vi "diffusion_sub.vi"(0 "X":dbl[](array[numeric]) format="%.2f", 1 "Standard Deviation":dbl[](array[numeric]) format="%.2f", 5 "Y":dbl[](array[numeric]) format="%.2f", 9 "Initial Guess Coefficients":dbl[](array[numeric])=[0.0, 1e-09, 0.0001, 0.8, 0.5] format="%.2e", 11 "max iteration":i32=200, 12 "Substitution Rules":T2(array[cluster])) -> (3 "Covariance":dbl[][](array[numeric]) format="%.2f", 4 "Best Fit Coefficients":dbl[](array[numeric]) format="%.2e", 6 "Best Fit":dbl[](array[numeric]) format="%.2f", 8 "ticks":i32=1, 10 "mse":dbl=nan format="%.2e", 14 "error":i32=-23033, 15 "model description":T1={"model"="b*(1+a*exp(-x/t1))/(1+x/t2)*(1+x/(4*t2))^(-1/2)+o", "Parameters"=["o", "t1", "t2", "b", "a"], "x"="x"})   [LabVIEW 2009]
uses:
  <vilib>/gmath/NI_Gmath.lvlib
panel:
  out "Parameters 4":string[](array[string])
  out "Best Fit Coefficients 2":dbl[](array[numeric]) format="%.2f"
  out "Parameters 3":string[](array[string])
  out "output array":dbl[](array[numeric]) format="%.2e"
  out "original par.":string[](array[string])
  out "Parameters":string[](array[string])
  out "error out":errorcluster
  # "Diffusion Fit\none component\none Triplet / chemical reaction\nvariable substituation"
  # "n:=1/b\nr:=a/(1+a)"
  # "b:=1/n\na:=r/(1-r)"
  # "1/n := b"
  # "r/(1-r) := a"
  # "k := 4"
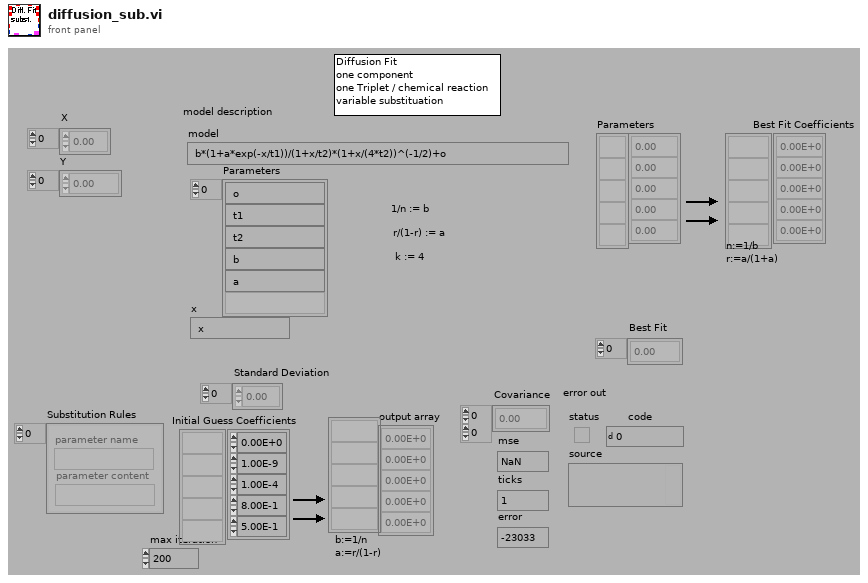
[diagram p1: front panel]
types:
  T1 = cluster{"model":string, "Parameters":string[], "x":string}
  T2 = cluster{"parameter name":string, "parameter content":string}[]
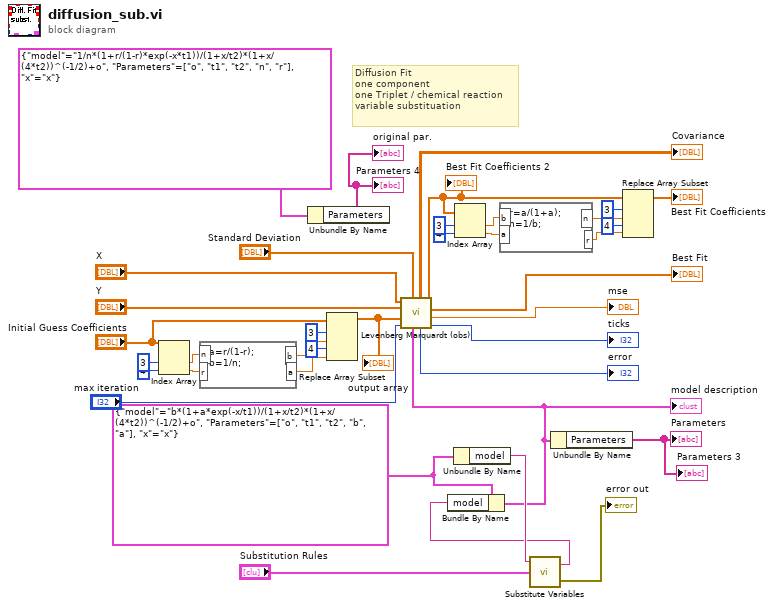
[diagram p0: block diagram]
diagram:
  w25 = T1 {"model"="b*(1+a*exp(-x/t1))/(1+x/t2)*(1+x/(4*t2))^(-1/2)+o", "Parameters"=["o", "t1", "t2", "b", "a"], "x"="x"} ("model description 2")
  # "just for show"
  # "Diffusion Fit\none component\none Triplet / chemical reaction\nvariable substituation"
  n1 = Index Array(array="Initial Guess Coefficients", index #1=3 ("index"), index #2=4 ("index")) -> (element #1=w17:dbl, element #2=w16:dbl)
  n2 = formula code="a=r/(1-r);\nb=1/n;"("n"=w17, "r"=w16) -> ("b"=w15:dbl, "a"=w14:dbl)
  n3 = Unbundle By Name(T1 {"model"="1/n*(1+r/(1-r)*exp(-x*t1))/(1+x/t2)*(1+x/(4*t2))^(-1/2)+o", "Parameters"=["o", "t1", "t2", "n", "r"], "x"="x"} ("model description 2")) -> ("Parameters"=→"original par." →"Parameters 4":string[])
  n4 = Replace Array Subset(array="Initial Guess Coefficients", new element #1=w15, index #1=3 ("index"), new element #2=w14, index #2=4 ("index")) -> (w4:dbl[])
  "output array" <- w4
  n5 = Unbundle By Name(w25) -> ("model"=w36:string)
  n6 = call "Substitute Variables.vi"("Substitution Rules"="Substitution Rules", "original formula"=w36) -> ("error out"=→"error out":errorcluster, "formula after substitution"=w26:string)  [unwired: 1 in]
  n7 = Bundle By Name(cluster=w25, "model"=w26) -> (w24:T1)
  "model description" <- w24
  n8 = call <vilib>:"Levenberg Marquardt (obs).vi"("model description"=w24, "Standard Deviation"="Standard Deviation", "max iteration"="max iteration", "Initial Guess Coefficient"=w4, "Y"="Y", "X"="X") -> ("ticks"=→"ticks":i32, "mse"=→"mse":dbl, "Best Fit"=→"Best Fit":dbl[], "Best Fit Coefficients"=w3:dbl[], "error"=→"error":i32, "Covariance"=→"Covariance":dbl[][])
  "Best Fit Coefficients 2" <- w3
  n9 = Index Array(array=w3, index #1=3 ("index"), index #2=4 ("index")) -> (element #1=w9:dbl, element #2=w8:dbl)
  n10 = formula code="r=a/(1+a);\nn=1/b;"("b"=w9, "a"=w8) -> ("n"=w7:dbl, "r"=w6:dbl)
  n11 = Unbundle By Name(w24) -> ("Parameters"=→"Parameters" →"Parameters 3":string[])
  n12 = Replace Array Subset(array=w3, new element #1=w7, index #1=3 ("index"), new element #2=w6, index #2=4 ("index")) -> (→"Best Fit Coefficients":dbl[])
